vi "q2 marks case structure.vi"() -> ()   [LabVIEW 2018]
panel:
  out "grade":string
  in  "marks":dbl
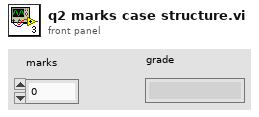
[diagram p1: front panel]
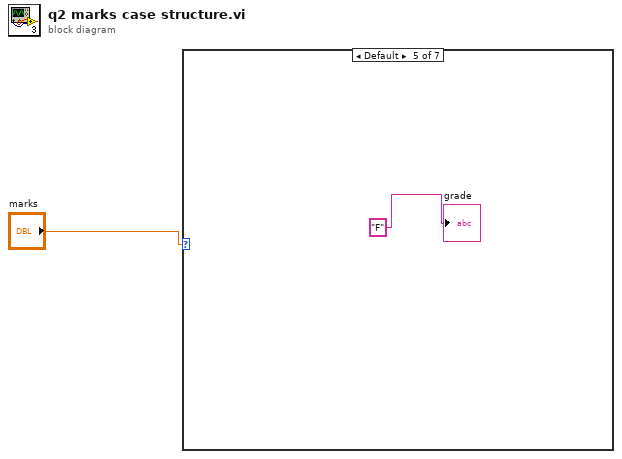
[diagram p0: block diagram]
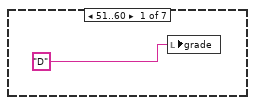
[diagram p2: hidden frame]
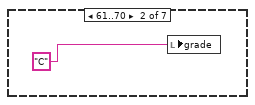
[diagram p3: hidden frame]
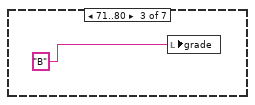
[diagram p4: hidden frame]
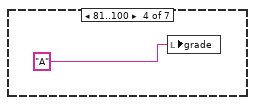
[diagram p5: hidden frame]
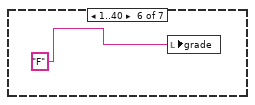
[diagram p6: hidden frame]
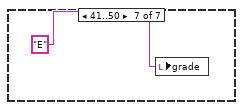
[diagram p7: hidden frame]
diagram:
  n1 = case shown="Default" "marks" {
    frame 51..60 {
      n2 = local write "grade"("D") -> ()
    }
    frame 61..70 {
      n3 = local write "grade"("C") -> ()
    }
    frame 71..80 {
      n4 = local write "grade"("B") -> ()
    }
    frame 81..100 {
      n5 = local write "grade"("A") -> ()
    }
    frame Default {
      "grade" <- "F"
    }
    frame 1..40 {
      n6 = local write "grade"("F") -> ()
    }
    frame 41..50 {
      n7 = local write "grade"("E") -> ()
    }
  }
